vi "Host - Thruster Update Cmd(SubVI).vi"(6 "Com":string[](array[string]), 8 "error in":errorcluster, 9 "IP Address":string[](array[string]), 10 "Serial Input":T1[](array[typedef])) -> (0 "error out":errorcluster, 2 "# elements in queue":i32)   [LabVIEW 2021]
uses:
  Async Serial/Controls/Async Frame Info Cluster.ctl
  Async Serial/Controls/Async Message Info Cluster.ctl
  Controls/Host Data Cluster.ctl
  Main Engine/Controls/Main Engine CPU Info.ctl
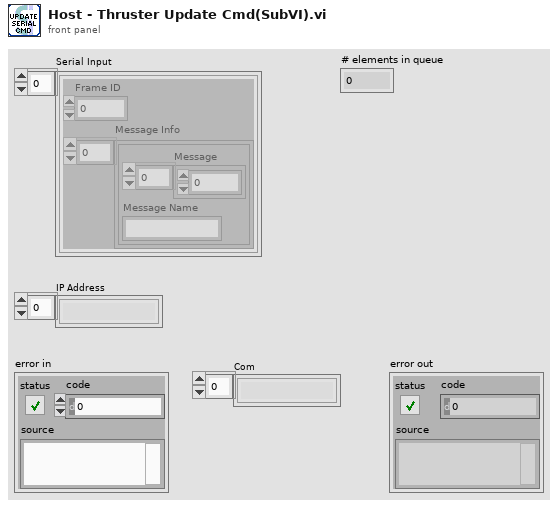
[diagram p1: front panel]
types:
  T1 = typedef "Async Frame Info Cluster.ctl" = cluster{"Frame ID":u16, "Message Info":T2[]}
  T2 = typedef "Async Message Info Cluster.ctl" = cluster{"Message":u8[], "Message Name":string}
  T3 = typedef "Host Data Cluster.ctl" = cluster{"AI":dbl[], "DI":bool[], "DO":bool[], "Serial":string[][], "CPU":T4, "Stop":bool, "DO Channel":string[]}
  T4 = typedef "Main Engine CPU Info.ctl" = cluster{"Total Load":u32[], "Interrupt Load":u32[], "Total Physical":dbl, "Free Physical":dbl, "Primary Disk Capacity":dbl, "Primary Disk Free":dbl}
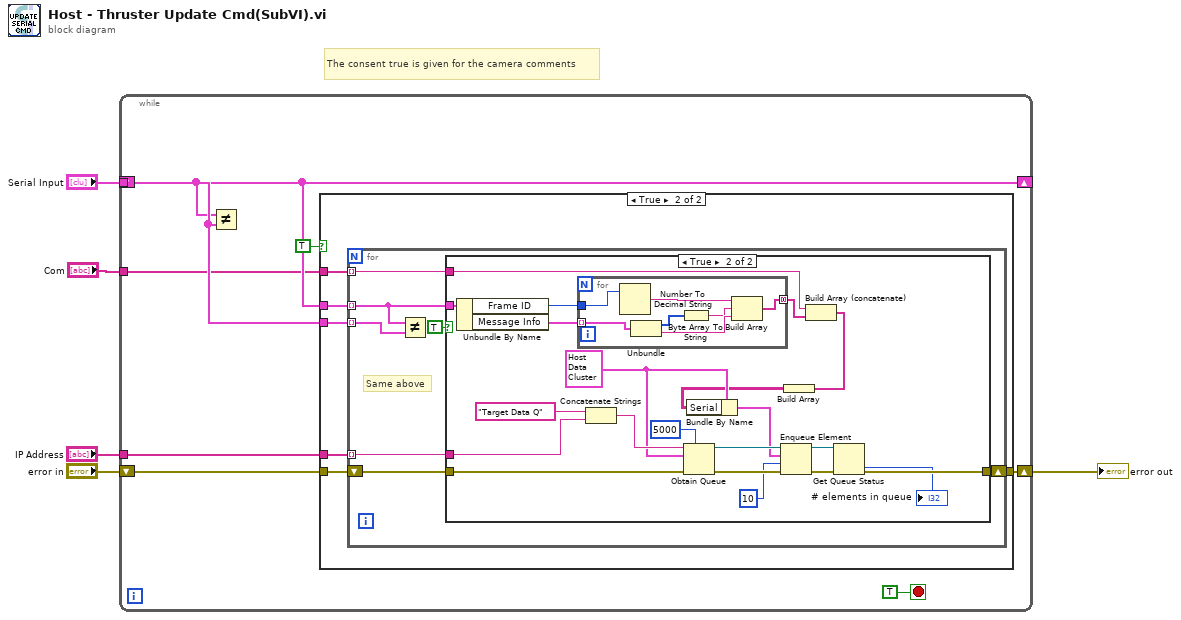
[diagram p0: block diagram]
diagram:
  # "The consent true is given for the camera comments"
  n1 = while {
    shift-right: [w8] -> _
    shift-left: _ -> [w9]
    tunnel: "Serial Input" -> [w8]
    shift-right: [w11] -> w5
    shift-left: "error in" -> [w12]
    tunnel: "IP Address" -> [w10]
    tunnel: "Com" -> [w7]
    stop <- TRUE stop-if-true
    n2 = Not Equal?(x=w8, y=w9) -> ()  [unwired: 1 out]
    n3 = case shown="True" TRUE {
      tunnel: w8 -> [_ w16]
      tunnel: w9 -> [_ w20]
      tunnel: w10 -> [_ w19]
      tunnel: w12 -> [w14 w18]
      tunnel: [w14 w17] -> w11
      tunnel: w7 -> [_ w15]
      frame False {
      }
      frame True {
        n4 = for {
          tunnel: w16 -> [w25] mode=indexing
          tunnel: w20 -> [w27] mode=indexing
          tunnel: w19 -> [w26] mode=indexing
          shift-right: [w23] -> w17
          shift-left: w18 -> [w24]
          tunnel: w15 -> [w22] mode=indexing
          # "Same above"
          n5 = Not Equal?(x=w25, y=w27) -> ()  [unwired: 1 out]
          n6 = case shown="True" TRUE {
            tunnel: w26 -> [_ w49]
            tunnel: w25 -> [_ w48]
            tunnel: w24 -> [w28 w47]
            tunnel: [w28 w31] -> w23
            tunnel: w22 -> [_ w33]
            frame False {
            }
            frame True {
              w42 = T3 {"AI"=[-3.29963760152739, -3.28042607250678, -3.30275742266883, -3.28305329003257, -3.29914499819412, -3.27566424083626, -3.29520417157553, -3.26269235518028, -3.14446761533159, -3.13215254239399, -3.16088771377303, -3.13198834142664, -3.16959036650255, -3.151528257494, -3.17188918049567, -3.1431540075152, -3.2208210848143, -3.21425304324317, -3.24479443847459, -3.23132995179905, -3.24922786722435, -3.22706072451644, -3.22311989941762, -3.18896608529332, -3.07895143597999, -3.07616002028715, -3.11064221681751, -3.08551947305428, -3.12459929803547, -3.10916440827463, -3.12197208267327], "DI"=[FALSE, FALSE, FALSE, FALSE, FALSE, FALSE, FALSE, FALSE, FALSE, FALSE, FALSE, FALSE, FALSE, FALSE, FALSE, FALSE, FALSE, FALSE, FALSE, FALSE, FALSE, FALSE, FALSE, FALSE, FALSE, FALSE, FALSE, FALSE, FALSE, FALSE, FALSE, FALSE, FALSE, FALSE, FALSE, FALSE, FALSE, FALSE, FALSE, FALSE, FALSE, FALSE, FALSE, FALSE, FALSE, FALSE, FALSE, FALSE, FALSE, FALSE, FALSE, FALSE, FALSE, FALSE, FALSE, FALSE, FALSE, FALSE, FALSE, FALSE, FALSE, FALSE, FALSE, FALSE], "DO"=[], "Serial"=[], "CPU"={"Total Load"=[], "Interrupt Load"=[], "Total Physical"=0.0, "Free Physical"=0.0, "Primary Disk Capacity"=0.0, "Primary Disk Free"=0.0}, "Stop"=FALSE, "DO Channel"=[]} ("Data Out")
              n7 = Unbundle By Name(w48) -> ("Frame ID"=w38:u16, "Message Info"=w37:T2[])
              n8 = for {
                tunnel: w38 -> [w56]
                tunnel: w37 -> [w53] mode=indexing
                tunnel: [w54] -> w36 mode=concatenating
                n9 = Number To Decimal String(number=w56) -> (decimal integer string=w55:string)  [unwired: 1 in]
                n10 = Unbundle(w53) -> ("Message"=w51:u8[], "Message Name"=w52:string)
                n11 = Byte Array To String(unsigned byte array=w51) -> (string=w50:string)
                n12 = Build Array(w55, w50, w52) -> (w54:string[])
              }
              n13 = Concatenate Strings("Target Data Q" ("name (unnamed)"), w49) -> (w46:string)
              n14 = Obtain Queue(max queue size (-1, unlimited)=5000, name (unnamed)=w46, element data type=w42, error in (no error)=w47) -> (queue out=w43:refnum<queue>, error out=w40:errorcluster)  [unwired: 1 in, 1 out]
              n15 = Build Array (concatenate)(w33, w36) -> (w35:string[])
              n16 = Build Array(w35) -> (w34:string[][])
              n17 = Bundle By Name(cluster=w42, "Serial"=w34) -> (w41:T3)
              n18 = Enqueue Element(queue=w43, element=w41, timeout in ms (-1)=10, error in (no error)=w40) -> (queue out=w29:refnum<queue>, error out=w32:errorcluster)  [unwired: 1 out]
              n19 = Get Queue Status(queue=w29, error in (no error)=w32) -> (error out=w31:errorcluster, # elements in queue=→"# elements in queue":i32)  [unwired: 1 in, 6 out]
            }
          }
        }
      }
    }
  }
  "error out" <- w5
